vi "Get Address Map Element.vi"(2 "tx core":refnum<class "niUSRP Tx Core v1 FPGA.lvclass">, 5 "index":u8) -> (6 "address map element":T1)   [LabVIEW 2025, in "niUSRP Tx Core v1 FPGA.lvclass"]
uses:
  niUSRP Tx Core v1 FPGA.lvclass
  <instrlib>/_niInstr/Instruction Framework/v1/FPGA/Typedefs/Address Map Element.ctl
  niUSRP Tx Core v1 FPGA.lvclass/niUSRP Tx Core v1 FPGA.ctl
  <instrlib>/_niInstr/Instruction Framework/v1/FPGA/Typedefs/niInstr Instruction Framework v1 FPGA.lvlib
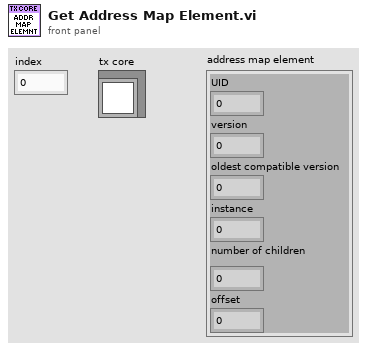
[diagram p1: front panel]
types:
  T1 = typedef "niInstr Instruction Framework v1 FPGA.lvlib/Address Map Element.ctl" = cluster{"UID":u16, "version":u16, "oldest compatible version":u16, "instance":u8, "number of children":u8, "offset":u32}
  T2 = typedef "niInstr Address Space Collection Builder v1 FPGA.lvlib/Parent Metadata.ctl" = cluster{"UID":u16, "version":u16, "oldest compatible version":u16}
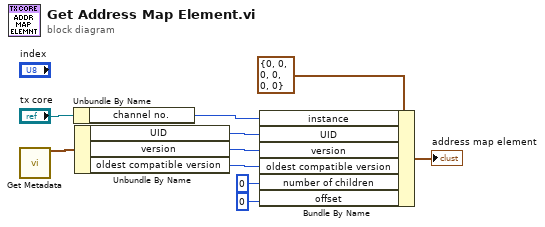
[diagram p0: block diagram]
diagram:
  n1 = call "Get Metadata.vi"() -> ("shared metadata"=w4:T2)  [unwired: 15 in]
  n2 = Unbundle By Name("tx core") -> ("channel no."=w5:u8)
  n3 = Unbundle By Name(w4) -> ("UID"=w3:u16, "version"=w2:u16, "oldest compatible version"=w1:u16)
  n4 = Bundle By Name(cluster=T1 {"UID"=0, "version"=0, "oldest compatible version"=0, "instance"=0, "number of children"=0, "offset"=0} ("address map element"), "instance"=w5, "UID"=w3, "version"=w2, "oldest compatible version"=w1, "number of children"=u8 0, "offset"=u32 0) -> (→"address map element":T1)
